vi "GetOneCtrlFromClusterCtrl.vi"(10 "index":u16, 11 "cluster":refnum<vi>) -> (3 "ctrl":refnum<vi>)   [LabVIEW 2018, in "Library-Ctrl.lvlib"]
uses:
  Library-Ctrl.lvlib
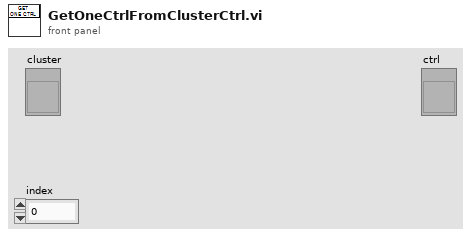
[diagram p1: front panel]
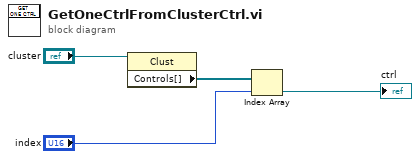
[diagram p0: block diagram]
diagram:
  n1 = property class="Clust"(reference="cluster") -> ("Controls[]"=w3:refnum<vi>[])  [unwired: 1 in, 2 out]
  n2 = Index Array(array=w3, index="index") -> (element=→"ctrl":refnum<vi>)
